vi "main_2 direction discrimination and data encoding.vi"() -> ()   [LabVIEW 2024]
doc: "This example shows how to configure multiple channels and acquire waveforms from multiple channels."
uses:
  RIGOL DS5000 7000 8000 Series/Public/Data/Read Waveform (Multiple).vi
  <vilib>/measure/mamon.llb/Waveform Peak Detection for 1 Chan.vi
  <vilib>/express/express analysis/Spectral/Block/exnSpectralBlock spectral measurements peak poly.vi
  <vilib>/express/express analysis/Spectral/Block/exnSpectralBlock spectral measurements peak WFM.vi
  <vilib>/Utility/file.llb/Write Delimited Spreadsheet (string).vi
  <vilib>/express/express analysis/Spectral/XNode/ExpressSpectralMeasurementsBlockNode.xnode
  RIGOL DS5000 7000 8000 Series/RIGOL DS5000 7000 8000 Series.lvlib
  <vilib>/measure/NI_MAPro.lvlib
panel:
  out "波形图表":dbl(graph)
  out "字符串":string
  in  "确定按钮":bool
  out "布尔 2":bool
  in  "Threshold":dbl=0.15
  in  "Save":bool
  out "Frequency":dbl
  in  "Time":dbl=20.0
  out "下拉列表":u16(ring)
  out "Count":dbl
  out "0, 1":i16
  out "子数组":dbl[](array[numeric])
  out "大小":i32
  out "# found":i32 caption="Count"
  in  "记时长度":dbl format="%#_13g"
  in  "Threshold":dbl=1.0
  out "Real time FFT":cluster{"f0":dbl, "df":dbl, "magnitude":dbl[]}(graph)
  out "输出数组":string[][](array[string])
  in  "停止":bool
  in  "Data format":string=".xls"
  in  "连接":bool
  in  "Data saving path":path
  in  "选项卡控件":enum32{"Channel 1", "Channel 2"}(tab)
  in  "Channel Number":u16(ring)=1 items=["Channel 1"=1, "Channel 2"=2]
  in  "电流方式":u16(ring)=1 items=["AC", "DC", "Ground"]
  in  "Probe Attenuation":u16(ring)=6 items=["0.01X", "0.02X", "0.05X", "0.1X", "0.2X", "0.5X", "1X", "2X", "5X", "10X", "20X", "50X", "100X", "200X", "500X", "1000X", "2000X", "5000X", "10000X", "20000X", "50000X"]
  in  "Time per Division (0.0005 s)":dbl=1e-07
  in  "Record Length (10k points)":u32=100000
  in  "Channel (2: Channel 2)":u16(ring)=2 items=["Channel 1"=1, "Channel 2"=2]
  in  "Vertical Coupling (1: DC)":u16(ring)=1 items=["AC", "DC", "Ground"]
  in  "Probe Attenuation  2":u16(ring)=6 items=["0.01X", "0.02X", "0.05X", "0.1X", "0.2X", "0.5X", "1X", "2X", "5X", "10X", "20X", "50X", "100X", "200X", "500X", "1000X", "2000X", "5000X", "10000X", "20000X", "50000X"]
  out "Received signal":waveform(dbl)[](graph)
  in  "Serial port":refnum<visa-resource-name>
  # "Chip-less Wireless Sensing System"
  # "Control panel"
  # "Count"
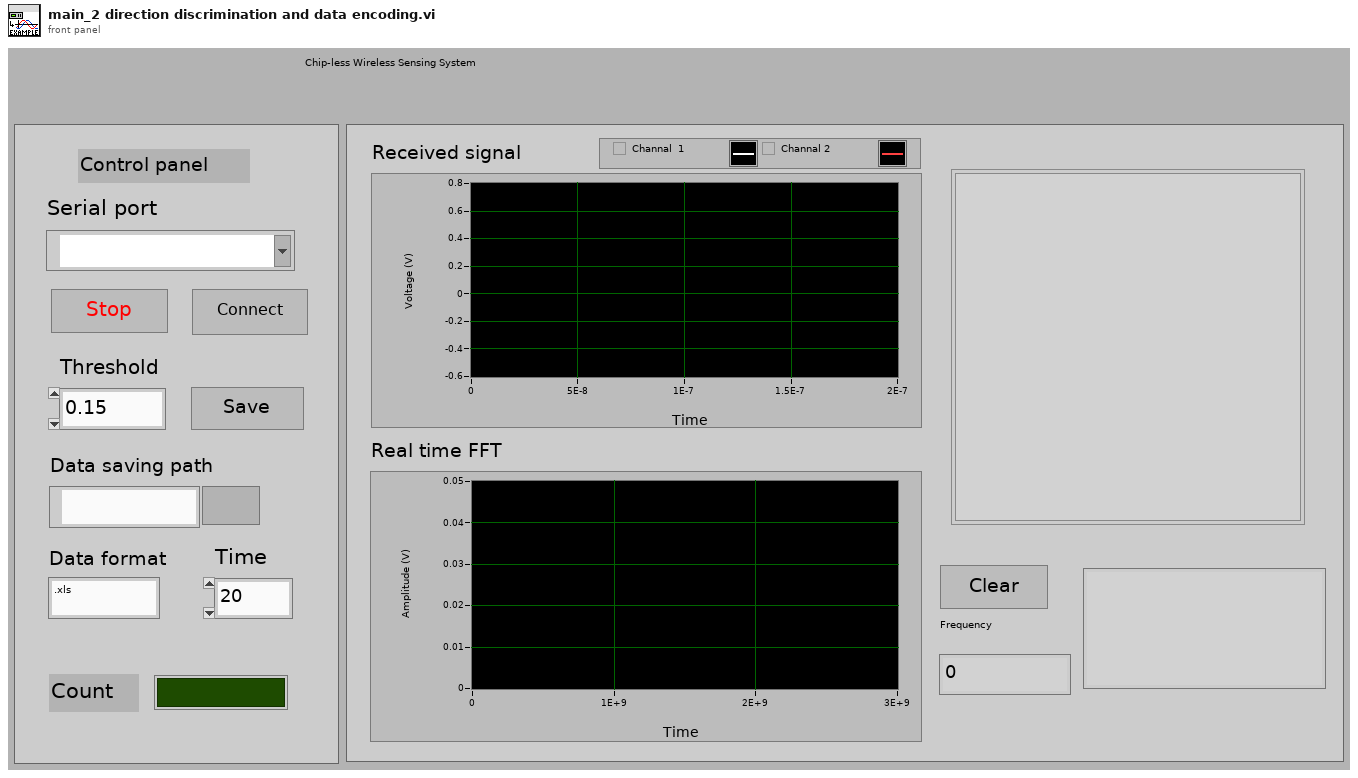
[diagram p1: front panel]
types:
  T1 = cluster{"averaging mode":u16, "weighting mode":u16, "number of averages":u32}
  T2 = cluster{"dB On (F)":bool, "unwrap phase (F)":bool, "convert to degree (F)":bool}
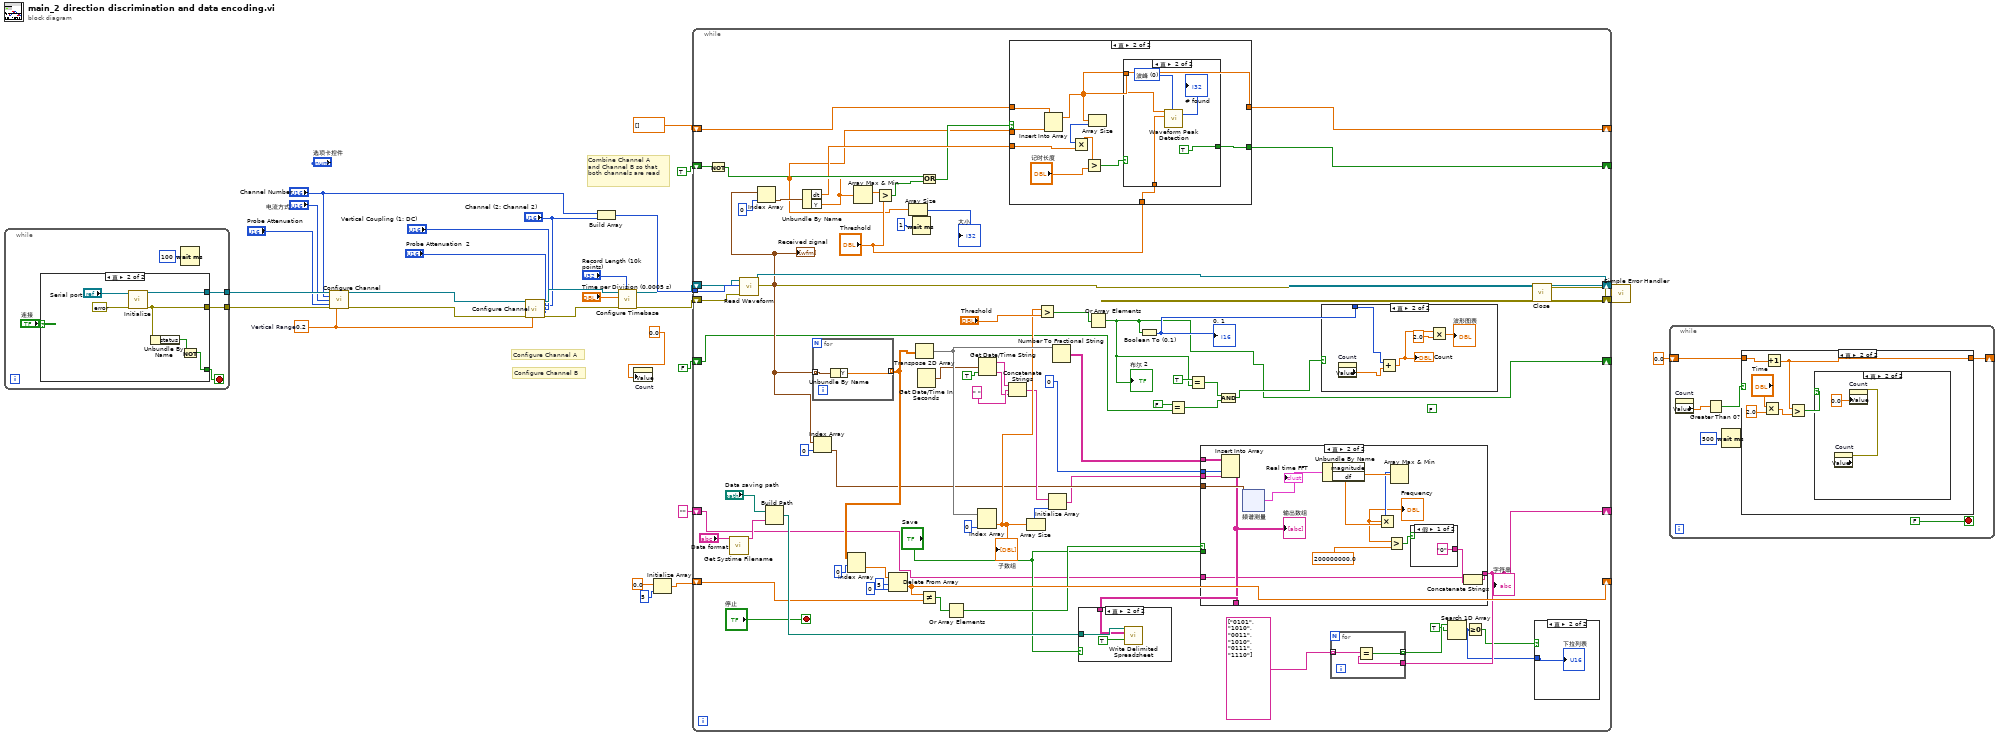
[diagram p0: block diagram]
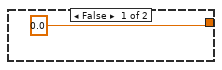
[diagram p2: hidden frame]
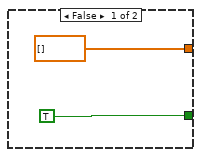
[diagram p6: hidden frame]
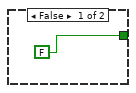
[diagram p7: hidden frame]
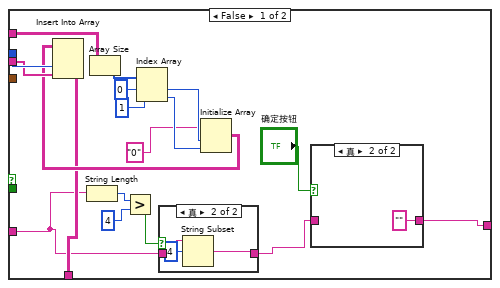
[diagram p9: hidden frame]
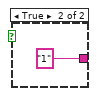
[diagram p12: hidden frame]
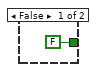
[diagram p13: hidden frame]
diagram:
  w23 = 0.2  # Vertical Range
  # "Combine Channel A\nand Channel B so that\nboth channels are read"
  # "Configure Channel B"
  # "Configure Channel A"
  n1 = while {
    tunnel: [w35] -> w29
    tunnel: [w34] -> w28
    stop <- w33 stop-if-true
    n2 = case shown="真" "连接" {
      tunnel: [_ w41] -> w35
      tunnel: [_ w39] -> w34
      tunnel: [FALSE w37] -> w33
      frame False {
      }
      frame True {
        n3 = call "Initialize.vi"("error in (no error)"=errorcluster {"status"=FALSE, "code"=0, "source"=""}, "VISA resource name"="Serial port") -> ("error out"=w39:errorcluster, "VISA resource name out"=w41:refnum<visa-resource-name>)  [unwired: 8 in]
        n4 = Unbundle By Name(w39) -> ("status"=w38:bool)
        n5 = Not(x=w38) -> (.not. x?=w37:bool)
      }
    }
    n6 = Wait (ms)(milliseconds to wait=u32 100 ("等待时间（毫秒）")) -> ()  [unwired: 1 out]
  }
  n7 = call "Configure Channel.vi"("VISA resource name"=w29, "Channel (1: Channel 1)"="Channel Number", "Vertical Coupling (1: DC)"="电流方式", "Probe Attenuation"="Probe Attenuation", "error in (no error)"=w28, "Vertical Range (10.0 V)"=w23) -> ("VISA resource name out"=w20:refnum<visa-resource-name>, "error out"=w19:errorcluster)  [unwired: 8 in]
  n8 = call "Configure Channel.vi"("VISA resource name"=w20, "Channel (1: Channel 1)"="Channel (2: Channel 2)", "Vertical Coupling (1: DC)"="Vertical Coupling (1: DC)", "Probe Attenuation"="Probe Attenuation  2", "error in (no error)"=w19, "Vertical Range (10.0 V)"=w23) -> ("VISA resource name out"=w27:refnum<visa-resource-name>, "error out"=w26:errorcluster)  [unwired: 8 in]
  n9 = Build Array("Channel Number", "Channel (2: Channel 2)") -> (w15:u16[])
  n10 = call "Configure Timebase.vi"("Record Length (10k points)"="Record Length (10k points)", "error in (no error)"=w26, "Time per Division (0.0005 s)"="Time per Division (0.0005 s)", "VISA resource name"=w27) -> ("error out"=w16:errorcluster, "VISA resource name out"=w14:refnum<visa-resource-name>)  [unwired: 6 in]
  n11 = property on="Count" class="DigNum (严格)"("Value"=0.0) -> ()  [unwired: 2 in, 2 out]
  n12 = Initialize Array(0.0, 5 ("维数大小")) -> (w7:dbl[])
  n13 = while {
    tunnel: w15 -> [w108]
    shift-right: [w110] -> w17
    shift-left: w16 -> [w109]
    shift-right: [w111] -> w18
    shift-left: w14 -> [w107]
    shift-right: [w83] -> _
    shift-left: w7 -> [w84]
    shift-right: [w66] -> _
    shift-left: dbl[] [] -> [w67]
    shift-right: [w63] -> _
    shift-left: TRUE -> [w69]
    shift-right: [w50] -> _
    shift-left: FALSE -> [w57]
    shift-right: [w48] -> _
    shift-left: "" -> [w43]
    stop <- "停止" stop-if-true
    (unwired) FALSE
    n14 = Not(x=w69) -> (.not. x?=w68:bool)
    n15 = call "Get Systime Filename.vi"("文件格式"="Data format") -> ("输出时间文件"=w104:string)  [unwired: 10 in]
    n16 = call-poly "Read Waveform.vi"("error in (no error)"=w109, "Channels"=w108, "VISA resource name"=w107) -> ("error out"=w110:errorcluster, "Waveform Data"=w74:waveform(dbl)[], "VISA resource name out"=w111:refnum<visa-resource-name>)  [unwired: 6 in]
    "Received signal" <- w74
    n17 = Index Array(array=w74, index=0 ("索引")) -> (element=w72:waveform(dbl))
    n18 = Build Path(base path="Data saving path", name or relative path=w104) -> (appended path=w103:path)
    n19 = Unbundle By Name(w72) -> ("dt"=w65:dbl, "Y"=w61:dbl[])
    n20 = for {
      tunnel: w74 -> [w194] mode=indexing
      tunnel: [w193] -> w89 mode=indexing
      n21 = Unbundle By Name(w194) -> ("Y"=w193:dbl[])
    }
    n22 = Index Array(array=w74, index=0 ("索引 (行)")) -> (element=w79:waveform(dbl))
    n23 = Index Array(array=w89, index (row)=0 ("索引 (行)")) -> (element=w87:dbl[])  [unwired: 1 in]
    n24 = Array Max & Min(array=w61) -> (max value=w71:dbl)  [unwired: 3 out]
    n25 = Greater?(x=w71, y="Threshold") -> (0:w70:bool)
    n26 = Delete From Array(array=w87, length=5 ("长度"), index=0 ("索引")) -> (deleted portion=w83:dbl[])  [unwired: 1 out]
    n27 = Array Size(array=w61) -> (size(s)=→"大小":i32)
    n28 = Wait (ms)(milliseconds to wait=u32 1 ("等待时间（毫秒）")) -> ()  [unwired: 1 out]
    n29 = Transpose 2D Array(2D array=w89) -> (transposed array=w101:dbl[][])
    n30 = Get Date/Time In Seconds() -> (seconds since 1Jan1904=w90:timestamp)
    n31 = Or(x=w68, y=w70) -> (x .or. y?=w64:bool)
    n32 = Not Equal?(x=w83, y=w84) -> (x != y?=w82:bool[])
    n33 = Or Array Elements(Boolean array=w82) -> (logical OR=w81:bool)
    n34 = Index Array(array=w101, index (col)=0 ("禁用的索引 (列)")) -> (element=w94:dbl[])  [unwired: 1 in]
    "子数组" <- w94
    n35 = Get Date/Time String(seconds (now)=w90, want seconds? (F)=TRUE ("需要秒？(F)")) -> (date string=w96:string, time string=w97:string)  [unwired: 1 in]
    n36 = Concatenate Strings(w96, " " ("字符串"), w97) -> (w93:string)
    n37 = case shown="真" w64 {
      tunnel: w61 -> [_ w132]
      tunnel: w67 -> [_ w131]
      tunnel: [dbl[] [] w124] -> w66
      tunnel: w65 -> [_ w129]
      tunnel: [TRUE w125] -> w63
      tunnel: "Threshold" -> [_ w123]
      frame False {
      }
      frame True {
        n38 = Insert Into Array(array=w131, new element=w132) -> (w124:dbl[])  [unwired: 1 in]
        n39 = Array Size(array=w124) -> (size(s)=w130:i32)
        n40 = Multiply(x=w130, y=w129) -> (x*y=w128:dbl)
        n41 = Greater?(x=w128, y="记时长度") -> (0:w126:bool)
        n42 = case shown="真" w126 {
          tunnel: [FALSE TRUE] -> w125
          tunnel: w124 -> [_ w137]
          tunnel: w123 -> [_ w136]
          frame False {
          }
          frame True {
            w135 = u16 0 items=["波峰", "波谷"] ("peaks/valleys")
            n43 = call-poly <vilib>:"Waveform Peak Detection.vi"("peaks/valleys"=w135, "threshold"=w136, "Signal In"=w137) -> ("# found"=→"# found":i32)  [unwired: 4 in, 4 out]
          }
        }
      }
    }
    n44 = Array Size(array=w94) -> (size(s)=w92:i32)
    n45 = Greater?(x=w94, y="Threshold") -> (0:w59:bool[])
    n46 = Initialize Array(w93, w92) -> (w75:string[])
    n47 = Number To Fractional String(number=w101) -> (F-format string=w77:string[][])  [unwired: 3 in]
    n48 = Or Array Elements(Boolean array=w59) -> (logical OR=w50:bool)
    "布尔 2" <- w50
    n49 = Boolean To (0,1)(Boolean=w50) -> (0, 1=w58:i16)
    "0, 1" <- w58
    n50 = Equal?(x=FALSE, y=w57) -> (x = y?=w53:bool)
    n51 = Equal?(x=TRUE, y=w50) -> (x = y?=w54:bool)
    n52 = case shown="真" w81 {
      tunnel: "Save" -> [_ _]
      tunnel: w79 -> [_ w180]
      tunnel: [w149 w176] -> w78
      tunnel: w77 -> [w151 w179]
      tunnel: 0 ("禁用的索引 (列)") -> [w153 w177]
      tunnel: w75 -> [w152 w178]
      tunnel: [w148 w167] -> w48
      tunnel: w43 -> [w143 w166]
      frame False {
        n53 = String Length(string=w143) -> (length=w146:i32)
        n54 = Array Size(array=w151) -> (size(s)=w159:i32[])
        n55 = Greater?(x=w146, y=4) -> (0:w144:bool)
        n56 = Index Array(array=w159, index #1=0 ("索引"), index #2=1 ("索引")) -> (element #1=w156:i32, element #2=w155:i32)
        n57 = case shown="真" w144 {
          tunnel: w143 -> [w160 w163]
          tunnel: [w160 w161] -> w142
          frame False {
          }
          frame True {
            n58 = String Subset(string=w163, offset (0)=4 ("偏移量(0)")) -> (substring=w161:string)  [unwired: 1 in]
          }
        }
        n59 = Initialize Array("0", w156, w155) -> (w150:string[][])
        n60 = Insert Into Array(array=w150, index (col)=w153, new element=w152) -> (w149:string[][])  [unwired: 1 in]
        n61 = case shown="真" "确定按钮" {
          tunnel: w142 -> [w164 _]
          tunnel: [w164 ""] -> w148
          frame False {
          }
          frame True {
          }
        }
      }
      frame True {
        n62 = Insert Into Array(array=w179, index (col)=w177, new element=w178) -> (w176:string[][])  [unwired: 1 in]
        "输出数组" <- w176
        n63 = xnode "频谱测量"("信号"=w180) -> ("FFT - （峰值）"=w175:cluster{"f0":dbl, "df":dbl, "magnitude":dbl[]})  [unwired: 1 in, 2 out]
        "Real time FFT" <- w175
        n64 = Unbundle By Name(w175) -> ("magnitude"=w174:dbl[], "df"=w172:dbl)
        n65 = Array Max & Min(array=w174) -> (max index (indices)=w173:i32)  [unwired: 3 out]
        n66 = Multiply(x=w173, y=w172) -> (x*y=w171:dbl)
        "Frequency" <- w171
        n67 = Greater?(x=w171, y=200000000.0) -> (0:w169:bool)
        n68 = case shown="假" w169 {
          tunnel: ["0" "1"] -> w168
          frame False {
          }
          frame True {
          }
        }
        n69 = Concatenate Strings(w166, w168) -> (w167:string)
      }
    }
    "字符串" <- w48
    n70 = case shown="真" "Save" {
      tunnel: w103 -> [_ w141]
      tunnel: w78 -> [_ w139]
      frame False {
      }
      frame True {
        n71 = call-poly <vilib>:"Write Delimited Spreadsheet.vi"("file path (dialog if empty)"=w141, "2D data"=w139, "append to file? (new file:F)"=TRUE) -> ()  [unwired: 11 in, 2 out]
      }
    }
    n72 = And(x=w54, y=w53) -> (x .and. y?=w52:bool)
    n73 = case shown="真" w52 {
      tunnel: w58 -> [_ w120]
      frame False {
      }
      frame True {
        n74 = property on="Count" class="DigNum (严格)"() -> ("Value"=w119:dbl)  [unwired: 2 in, 2 out]
        n75 = Add(x=w120, y=w119) -> (x+y=w118:dbl)
        "Count" <- w118
        n76 = Multiply(x=w118, y=2.0) -> (x*y=→"波形图表":dbl)
      }
    }
    n77 = for {
      tunnel: string[] ["0101", "1010", "0011", "1010", "0111", "1110"] -> [w115] mode=indexing
      tunnel: w48 -> [w114]
      tunnel: [w113] -> w47 mode=indexing
      n78 = Equal?(x=w115, y=w114) -> (x = y?=w113:bool)
    }
    n79 = Search 1D Array(1D array=w47, element=TRUE ("元素")) -> (index of element=w44:i32)  [unwired: 1 in]
    n80 = Greater Or Equal To 0?(x=w44) -> (x >= 0?=w45:bool)
    n81 = case shown="真" w45 {
      tunnel: w44 -> [_ w112]
      frame False {
      }
      frame True {
        "下拉列表" <- w112
      }
    }
  }
  n82 = call "Close.vi"("error in (no error)"=w17, "VISA resource name"=w18) -> ("error out"=w30:errorcluster)  [unwired: 9 in]
  n83 = call <vilib>:"Simple Error Handler.vi"("error in (no error)"=w30) -> ()  [unwired: 4 in, 5 out]
  n84 = while {
    shift-right: [w196] -> _
    shift-left: 0.0 -> [w197]
    stop <- FALSE stop-if-true
    n85 = property on="Count" class="DigNum (严格)"() -> ("Value"=w199:dbl)  [unwired: 2 in, 2 out]
    n86 = Greater Than 0?(x=w199) -> (x > 0?=w198:bool)
    n87 = Wait (ms)(milliseconds to wait=u32 500 ("等待时间（毫秒）")) -> ()  [unwired: 1 out]
    n88 = case shown="真" w198 {
      tunnel: w197 -> [_ w207]
      tunnel: [0.0 w206] -> w196
      frame False {
      }
      frame True {
        n89 = Multiply(x="Time", y=2.0) -> (x*y=w205:dbl)
        n90 = Increment(x=w207) -> (x+1=w206:dbl)
        n91 = Greater?(x=w206, y=w205) -> (0:w202:bool)
        n92 = case shown="真" w202 {
          frame False {
          }
          frame True {
            n93 = property on="Count" class="DigNum (严格)" props=["Value"]() -> (error out=w208:errorcluster)  [unwired: 2 in, 2 out]
            n94 = property on="Count" class="DigNum (严格)"(error in=w208, "Value"=0.0 ("震荡计数")) -> ()  [unwired: 1 in, 2 out]
          }
        }
      }
    }
  }
